vi "Clousure.vi"(8 "error in (no error)":errorcluster, 11 "Maze":refnum<class "Maze.lvclass">) -> (0 "error out":errorcluster, 3 "Maze":refnum<class "Maze.lvclass">)   [LabVIEW 2020, in "Maze.lvclass"]
uses:
  Maze.lvclass
  Maze.lvclass/Maze.ctl
  Private/Property/mRoomVec/Read mRoomVec.vi
  ConcreteMazeSite/Room/Room.lvclass
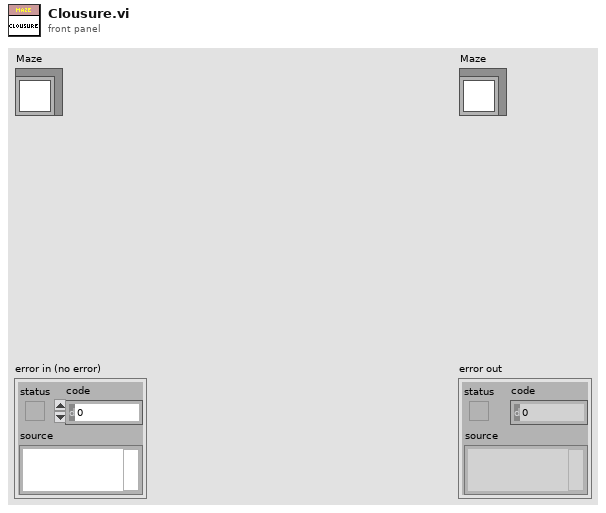
[diagram p1: front panel]
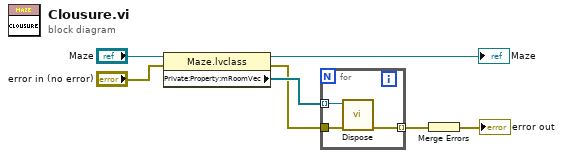
[diagram p0: block diagram]
diagram:
  n1 = property class="Maze.lvclass"(reference="Maze", error in="error in (no error)") -> (reference out=→"Maze":refnum<class "Maze.lvclass">, error out=w4:errorcluster, "Private:Property:mRoomVec"=w5:refnum<class "Room.lvclass">[])
  n2 = for {
    tunnel: w5 -> [w10] mode=indexing
    tunnel: w4 -> [w9]
    tunnel: [w8] -> w3 mode=indexing
    n3 = call-dynamic "Dispose.vi"("error in (no error)"=w9, "Room"=w10) -> ("error out"=w8:errorcluster)  [unwired: 9 in]
  }
  n4 = Merge Errors(w3) -> (→"error out":errorcluster)
